vi "Set_Active_Device.vi"(8 "error in (no error)":errorcluster, 10 "device":T1) -> (0 "error out":errorcluster)   [LabVIEW 2019, in "Kinova MICO² USB.lvlib"]
uses:
  <vilib>/Utility/error.llb/Error Cluster From Error Code.vi
  <vilib>/ErrorRing/Error Ring.xnode
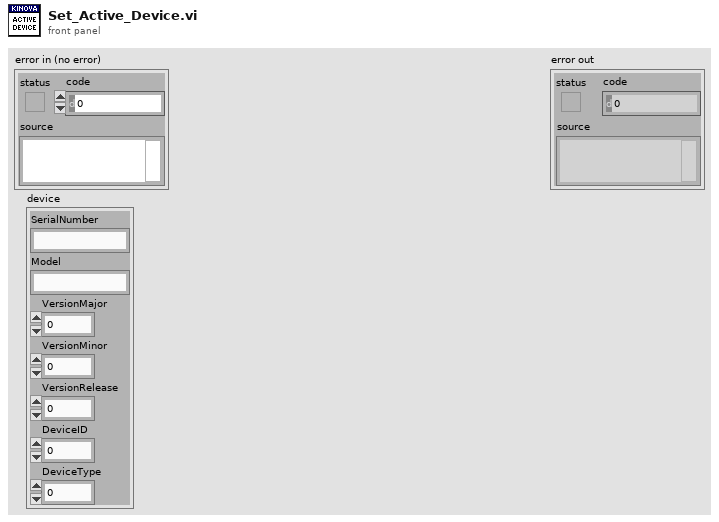
[diagram p1: front panel]
types:
  T1 = cluster{"SerialNumber":string, "Model":string, "VersionMajor":i32, "VersionMinor":i32, "VersionRelease":i32, "DeviceID":i32, "DeviceType":i32}
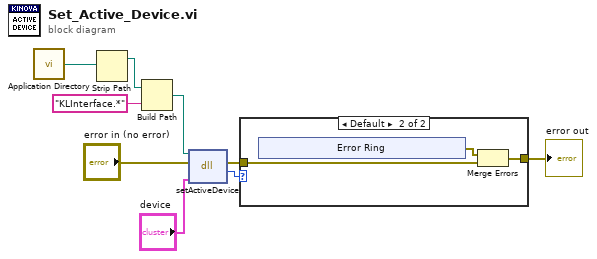
[diagram p0: block diagram]
diagram:
  n1 = call <vilib>:"Application Directory.vi"() -> ("Application Directory"=w1:path)
  n2 = Strip Path(path=w1) -> (stripped path=w8:path)  [unwired: 1 out]
  n3 = Build Path(base path=w8, name or relative path="KLInterface.*") -> (appended path=w2:path)
  n4 = dll-call lib="C:/Users/mcjssdcc/source/repos/Kinova Labview Interface/Debug/KLInterface.dll" fn="setActiveDevice"(path in=w2, error in="error in (no error)", "device"="device") -> (error out=w5:errorcluster, "return type"=w4:i32)  [unwired: 2 in, 1 out]
  n5 = case shown="Default" w4 {
    tunnel: [w10 w12] -> w7
    tunnel: w5 -> [w10 w11]
    frame 1 {
    }
    frame Default {
      n6 = xnode "Error Ring"() -> ("error out"=w13:errorcluster)
      n7 = Merge Errors(w13, w11) -> (w12:errorcluster)
    }
  }
  "error out" <- w7
